vi "itc Hg box controller -- Pgg2.vi"(6 "Log File Path":path, 7 "itc box action":T8=enum."init", 8 "error in":errorcluster, 9 "Sweep Table In":dbl[][](array[numeric])=[[650.0, 1334.0, 30.0], [300.0, 1334.0, 0.0], [0.0, 0.0, 0.0], [0.0, 0.0, 0.0], [0.0, 0.0, 0.0], [0.0, 0.0, 0.0], [0.0, 0.0, 0.0], [0.0, 0.0, 0.0], [0.0, 0.0, 0.0], [0.0, 0.0, 0.0], [0.0, 0.0, 0.0], [300.0, 0.0, 0.0], [0.0, 0.0, 0.0], [0.0, 0.0, 0.0], [0.0, 0.0, 0.0], [300.0, 0.0, 0.0]], 10 "input":dbl=10.0, 11 "VISA resource name":refnum<visa-resource-name>="GPIB0::1::INSTR") -> (0 "error out":errorcluster, 1 "Sweep Table":dbl[][](array[numeric])=[[650.0, 1334.0, 30.0], [300.0, 1334.0, 0.0], [0.0, 0.0, 0.0], [0.0, 0.0, 0.0], [0.0, 0.0, 0.0], [0.0, 0.0, 0.0], [0.0, 0.0, 0.0], [0.0, 0.0, 0.0], [0.0, 0.0, 0.0], [0.0, 0.0, 0.0], [0.0, 0.0, 0.0], [300.0, 0.0, 0.0], [0.0, 0.0, 0.0], [0.0, 0.0, 0.0], [0.0, 0.0, 0.0], [300.0, 0.0, 0.0]], 2 "itc box state OUT":T7={"ITC503 Address"="GPIB0::15::INSTR", "ITC temperature"=0.0, "ITC set temperature"=300.0, "heater"=300.0, "gas flow"=1.6, "P"=0.0, "D"=10.0, "I"=0.1, "ITC state"="X0A1C2S01H1L0\r", "nonzero temperature"=0.0, "Magn Field (T)"=0.0})   [LabVIEW 2015]
uses:
  itc 503 box - control.ctl
  itc 503 box state.ctl
  mercury ixx/public/libraries/auxiliary/Controls/AUX Device (Set).ctl
  mercury ixx/public/libraries/auxiliary/Controls/AUX Signals (Set).ctl
  mercury ixx/public/libraries/auxiliary/Controls/AUX Device (Read).ctl
  mercury ixx/public/Controls/Manufacturing Data.ctl
  mercury ixx/public/libraries/auxiliary/Controls/AUX Signals (Read).ctl
  mercury ixx/public/Controls/ISOBus Address.ctl
  mercury ixx/public/Controls/Comms Transport Layer.ctl
  comparison control.ctl
  mercury ixx/public/Controls/Unit String.ctl
  mercury ixx/public/libraries/heater/Controls/Heater Device (Set).ctl
  mercury ixx/public/libraries/heater/Controls/Heater Signals Cluster.ctl
  Q - not nan -- real.vi
  mercury ixx/public/libraries/auxiliary/Open/Open Auxiliary Device.vi
  mercury ixx/public/libraries/auxiliary/configuration/Read/Aux Device (Read).vi
  mercury ixx/public/libraries/auxiliary/configuration/Set/Aux Device (Set).vi
  mercury ixx/public/libraries/Temperature/Open/Open Temperature Device.vi
  mercury ixx/public/libraries/Temperature/Configuration/Read/Temperature Device (Read).vi
  mercury ixx/public/libraries/control loop/configuration/Set/Temperature Setpoint (Set).vi
  mercury ixx/public/libraries/control loop/configuration/Set/P Value (Set).vi
  mercury ixx/public/libraries/control loop/configuration/Set/I Value (Set).vi
  mercury ixx/public/libraries/control loop/configuration/Set/D Value (Set).vi
  mercury ixx/public/libraries/control loop/configuration/Set/Heater Auto (Set).vi
  mercury ixx/public/libraries/heater/Open/Open Heater Device.vi
  mercury ixx/public/libraries/heater/Configuration/Read/Heater Device (Read).vi
  mercury ixx/public/libraries/heater/Configuration/Set/Heater Device (Set).vi
  mercury ixx/public/libraries/control loop/configuration/Read/Temperature Setpoint (Read).vi
  mercury ixx/public/libraries/control loop/configuration/Read/PID (Read).vi
  mercury ixx/public/libraries/heater/signals/Read/Voltage (Read).vi
  mercury ixx/public/libraries/System.lvlib
  mercury ixx/Mercury iXX.lvlib
  mercury ixx/public/libraries/Auxiliary.lvlib
  mercury ixx/public/libraries/Temperature.lvlib
  mercury ixx/public/libraries/Control Loop.lvlib
  mercury ixx/public/libraries/Heater.lvlib
panel:
  out "Tab Control":T1(tab)
  out "Auxiliary Device OUT":T2 {"Signals"."% Open" min=0.0 max=100.0 step=0.1 format="%.4f"; "Signals"."Position" max=20.0 step=1.0 format="%.4f"; "Speed" max=7 step=1; "Gear" max=7 step=1; "Temp V Err" min=0.0 max=20.0 step=0.1; "Temp Err" min=0.0 max=20.0 step=0.1; "Scaling Factor" min=0.0 max=99.0 step=0.1; "Min Flow" min=0.0 max=20.0 step=0.1}
  in  "Auxiliary Device IN":T5 {"Signals"."% Open" min=0.0 max=100.0 step=0.1 format="%#.1f"; "Speed" max=7 step=1; "Gear" max=7 step=1; "Temp V Err" min=0.0 max=20.0 step=0.1; "Temp Err" min=0.0 max=20.0 step=0.1; "Scaling Factor" min=0.0 max=99.0 step=0.1; "Min Flow" min=0.0 max=20.0 step=0.1}
  out "enabled state":enum16{"disabled", "enabled"}(ring)
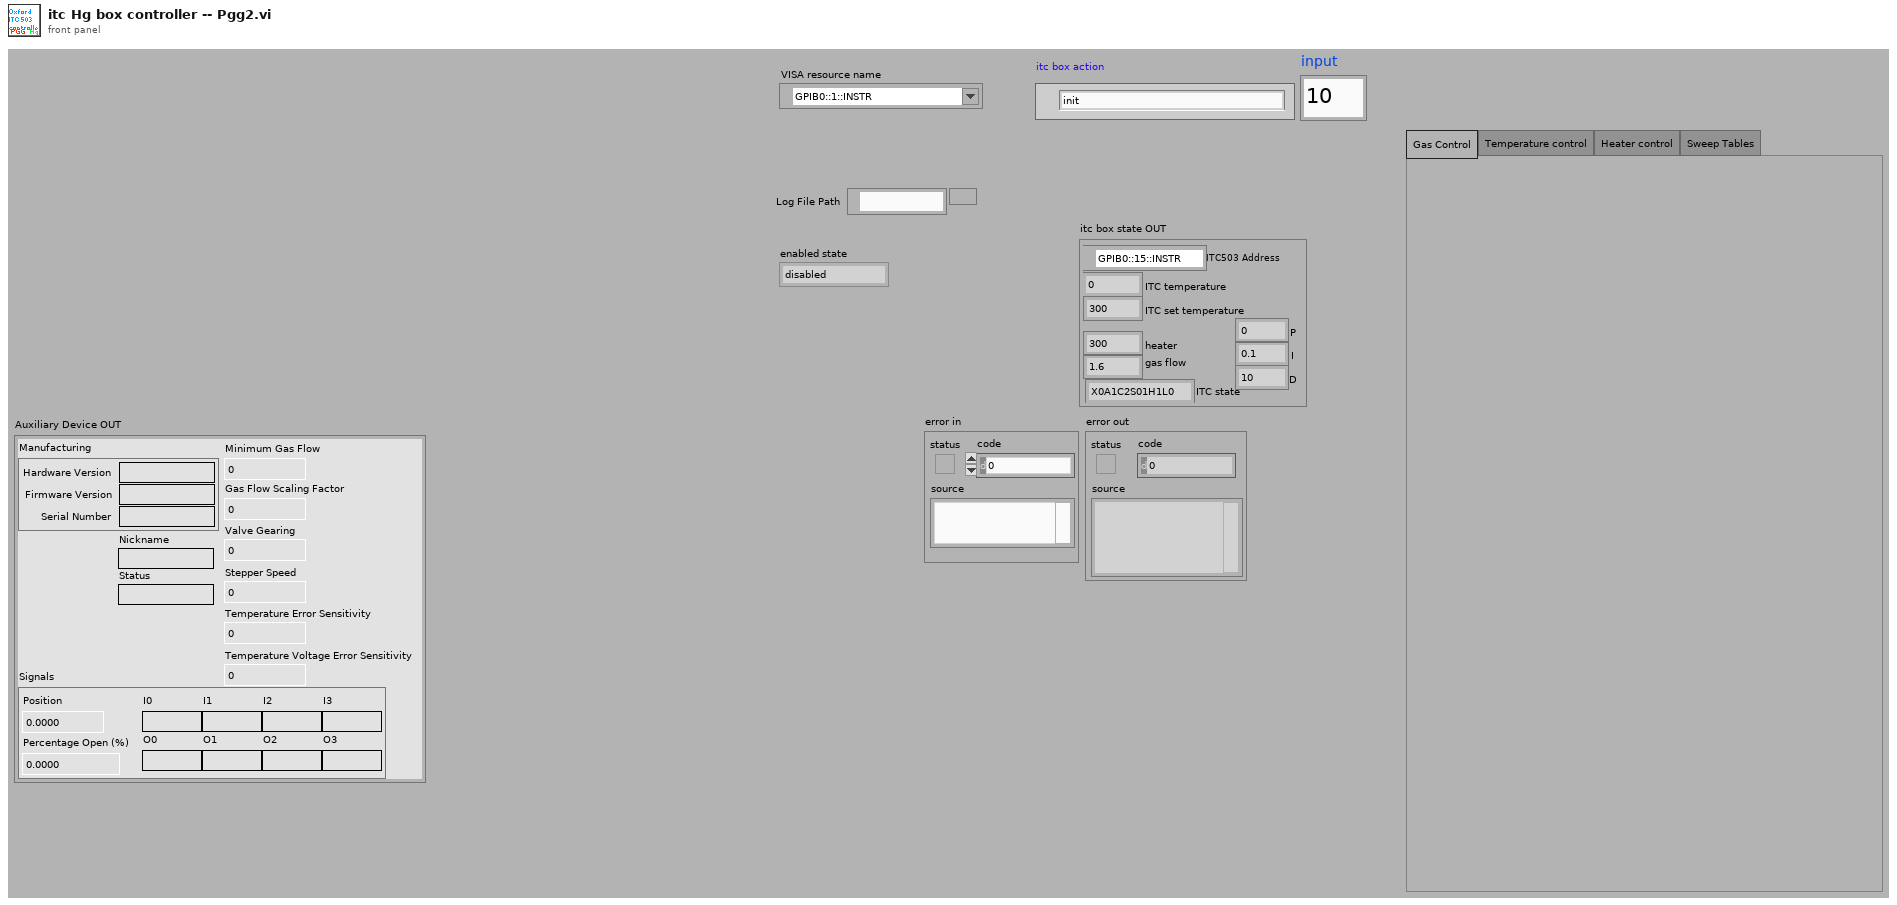
[diagram p1: front panel]
types:
  T1 = enum32{"Gas Control", "Temperature control", "Heater control", "Sweep Tables"}
  T2 = typedef "Mercury iXX.lvlib/Auxiliary.lvlib/AUX Device (Read).ctl" = cluster{"Manufacturing":T3, "Min Flow":dbl, "Scaling Factor":dbl, "Temp Err":dbl, "Temp V Err":dbl, "Gear":u32, "Speed":u32, "Signals":T4, "Nickname":string, "Status":string}
  T3 = typedef "Mercury iXX.lvlib/Manufacturing Data.ctl" = cluster{"Hardware Version":string, "Firmware Version":string, "Serial Number":string}
  T4 = typedef "Mercury iXX.lvlib/Auxiliary.lvlib/AUX Signals (Read).ctl" = cluster{"Position":dbl, "% Open":dbl, "I0":string, "I1":string, "I2":string, "I3":string, "O0":string, "O1":string, "O2":string, "O3":string}
  T5 = typedef "Mercury iXX.lvlib/Auxiliary.lvlib/AUX Device (Set).ctl" = cluster{"Min Flow":dbl, "Scaling Factor":dbl, "Temp Err":dbl, "Temp V Err":dbl, "Gear":u32, "Speed":u32, "Signals":T6}
  T6 = typedef "Mercury iXX.lvlib/Auxiliary.lvlib/AUX Signals (Set).ctl" = cluster{"% Open":dbl}
  T7 = typedef "itc 503 box state.ctl" = cluster{"ITC503 Address":refnum<visa-resource-name>, "ITC temperature":dbl, "ITC set temperature":dbl, "heater":dbl, "gas flow":dbl, "P":dbl, "D":dbl, "I":dbl, "ITC state":string, "nonzero temperature":dbl, "Magn Field (T)":dbl}
  T8 = typedef "itc 503 box - control.ctl" = enum16{"heater manual and zero", "heater auto", "upload D", "upload I", "upload P", "shut off", "init", "read sweep table", "disable", "enable", "read state", "set gas to", "stop sweep", "start sweep", "test", "set temperature to", "write sweep table", "-void", "set heater to"}
  T9 = typedef "Mercury iXX.lvlib/ISOBus Address.ctl" = i32
  T10 = typedef "Mercury iXX.lvlib/Comms Transport Layer.ctl" = enum16{"Ethernet TCP/IP", "USB", "ISOBus - RS-232", "GPIB"}
  T11 = typedef "Mercury iXX.lvlib/Unit String.ctl" = string
  T12 = typedef "Mercury iXX.lvlib/Heater.lvlib/Heater Device (Set).ctl" = cluster{"Nickname":string, "Voltage Limit":string, "Nominal Resistance":string, "Maximum Power":string, "Heater Signals":T13}
  T13 = typedef "Mercury iXX.lvlib/Heater.lvlib/Heater Signals Cluster.ctl" = cluster{"Voltage":string, "Current":string, "Power":string}
  T14 = typedef "Mercury iXX.lvlib/Mercury Reference.ctl" = cluster{"Comms":refnum<visa-resource-name>, "Device ID":string[], "Comms Layer":T10, "Command":string, "Query reference":T15}
  T15 = typedef "Mercury iXX.lvlib/Query Dynamic Reference.ctl" = refnum<vi>
  T16 = typedef "comparison control.ctl" = enum16{"not a number", "above", "in range", "below"}
  T17 = typedef "Mercury iXX.lvlib/Heater.lvlib/Heater Device (Read).ctl" = cluster{"Manufacturing":T3, "Nickname":string, "Voltage Limit":string, "Nominal Resistance":string, "Maximum Power":string, "Heater Signals":T13, "Status":string}
  T18 = typedef "Mercury iXX.lvlib/Control Loop.lvlib/PID cluster.ctl" = cluster{"P":dbl, "I":dbl, "D":dbl}
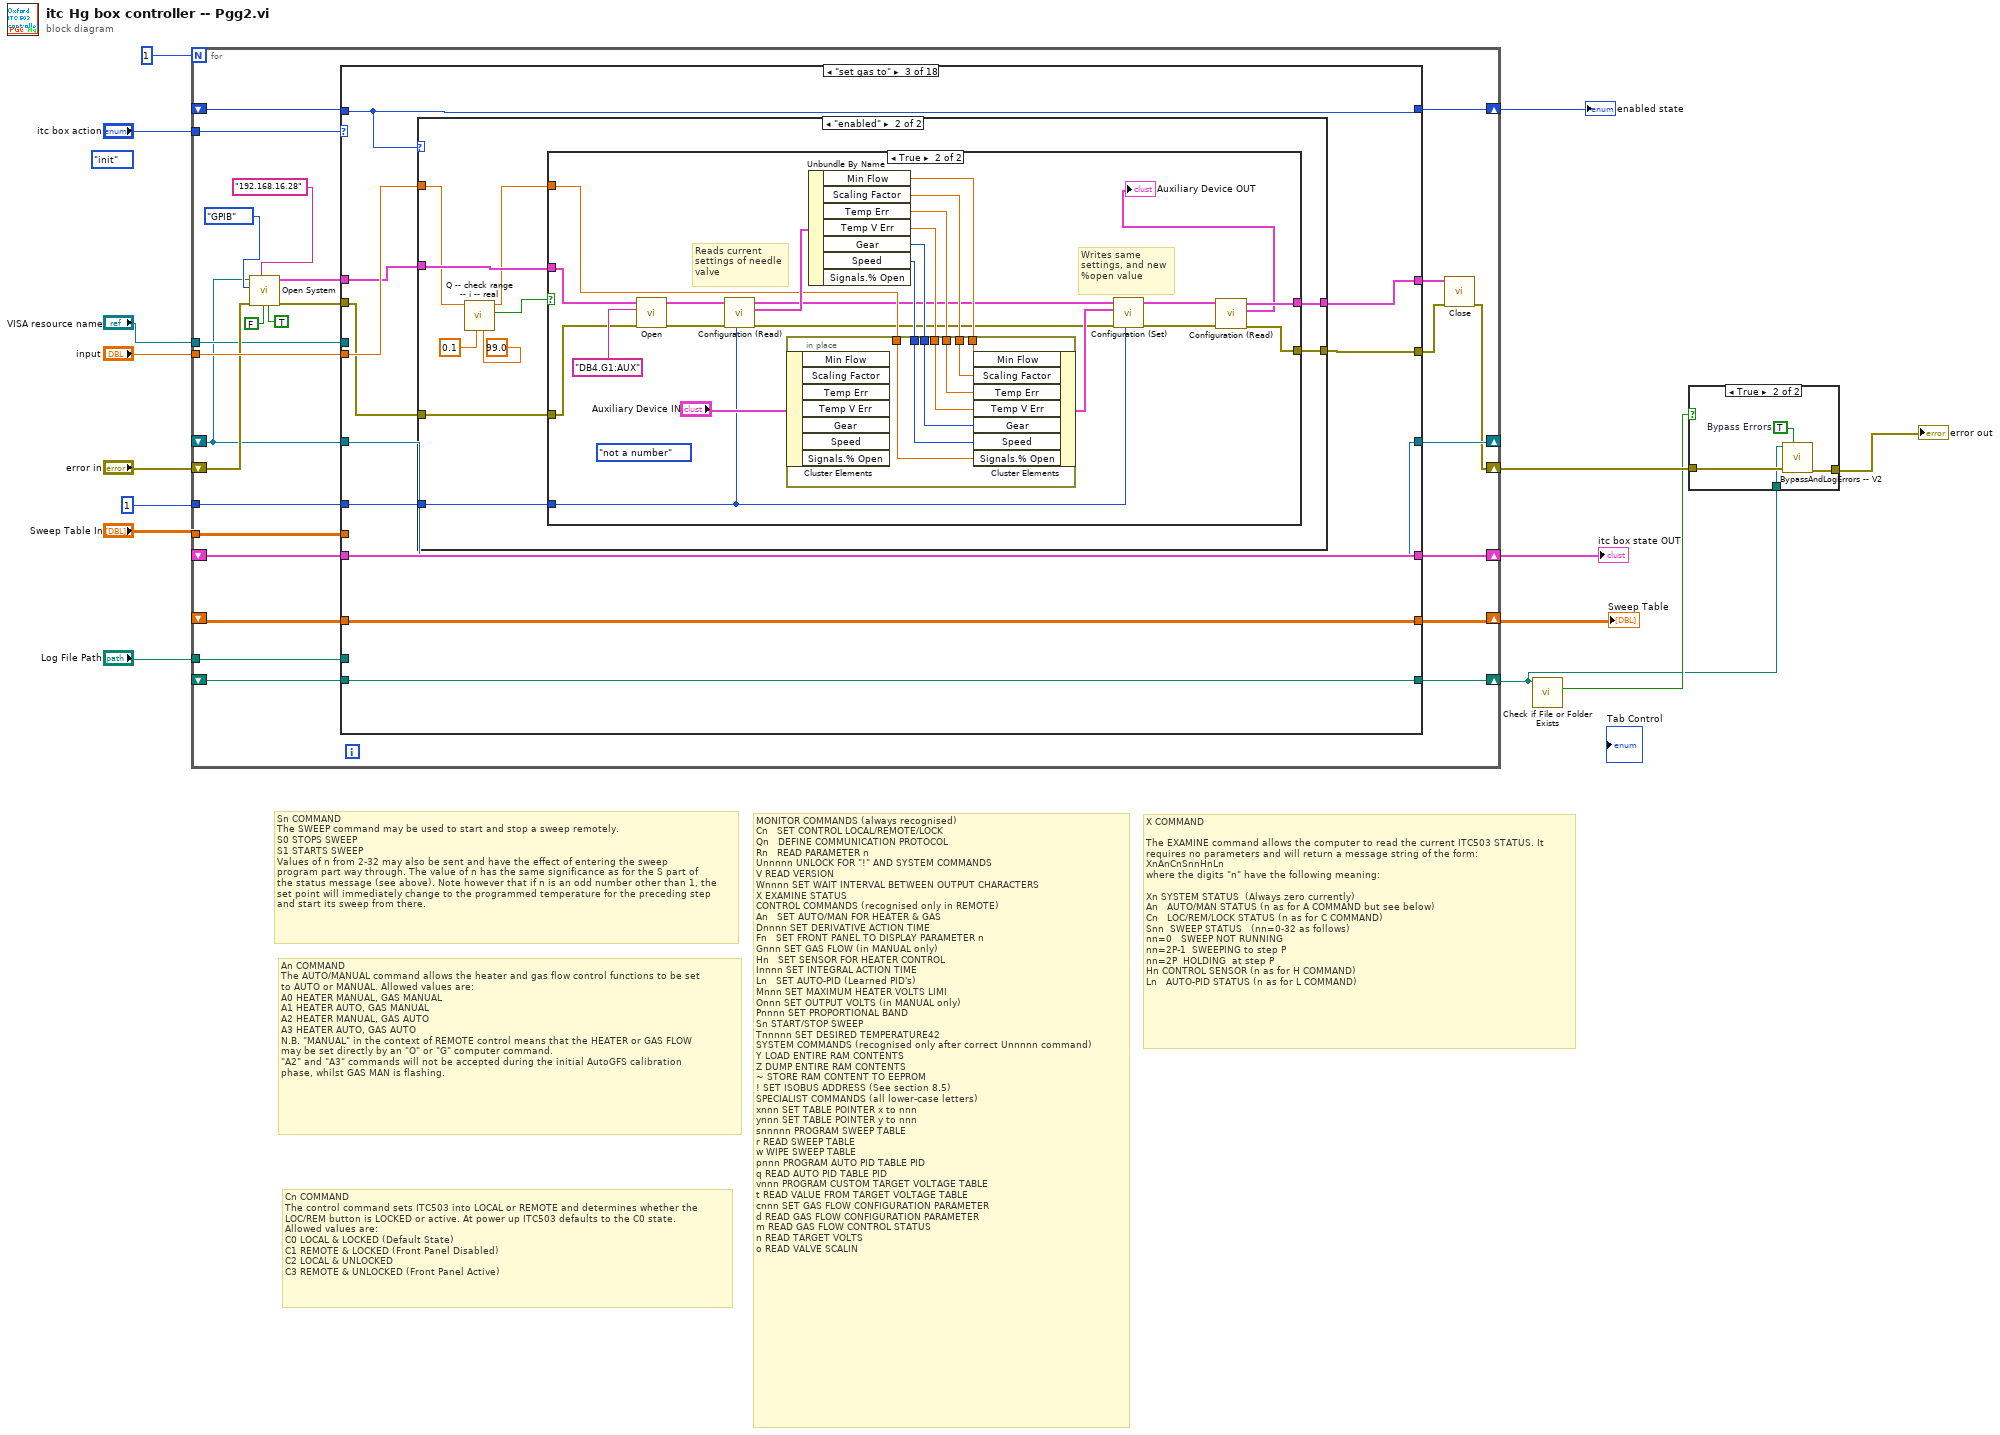
[diagram p0: block diagram]
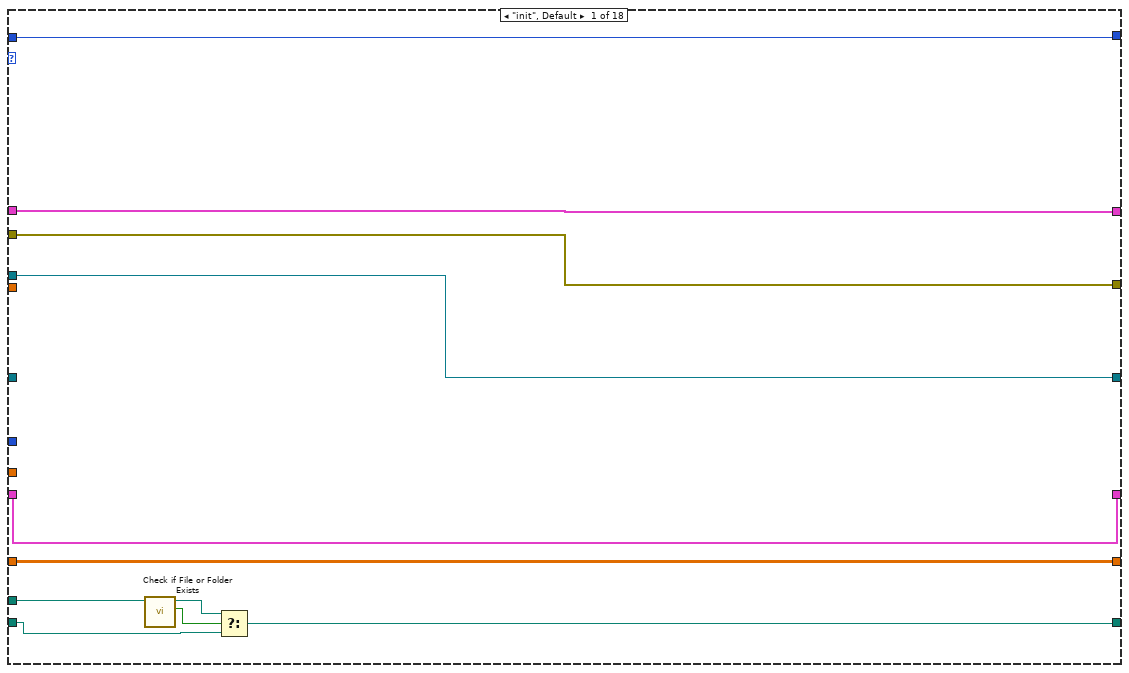
[diagram p3: hidden frame]
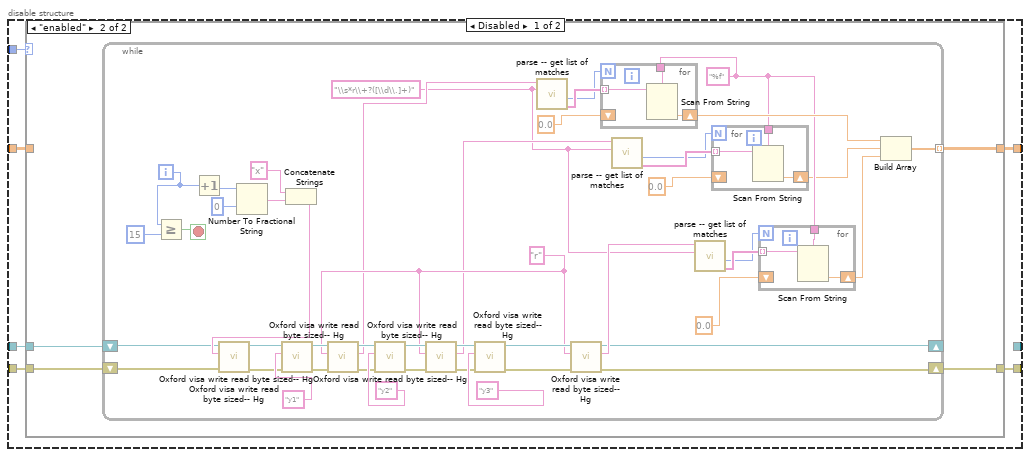
[diagram p5: hidden frame]
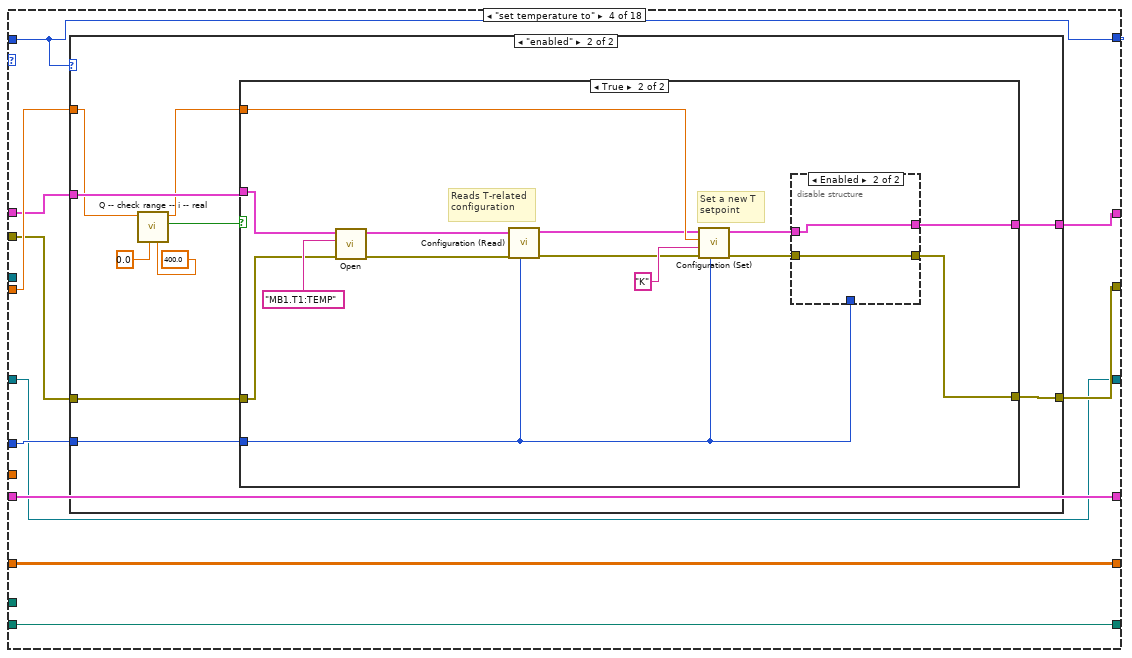
[diagram p9: hidden frame]
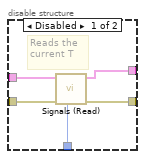
[diagram p12: hidden frame]
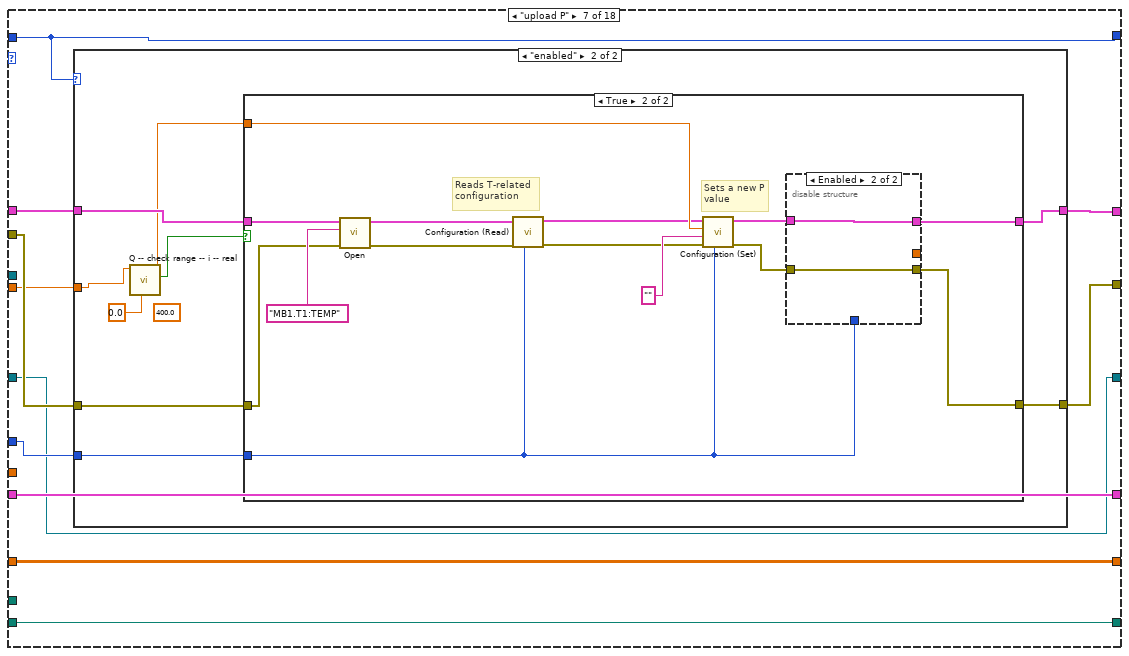
[diagram p15: hidden frame]
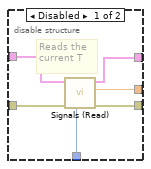
[diagram p18: hidden frame]
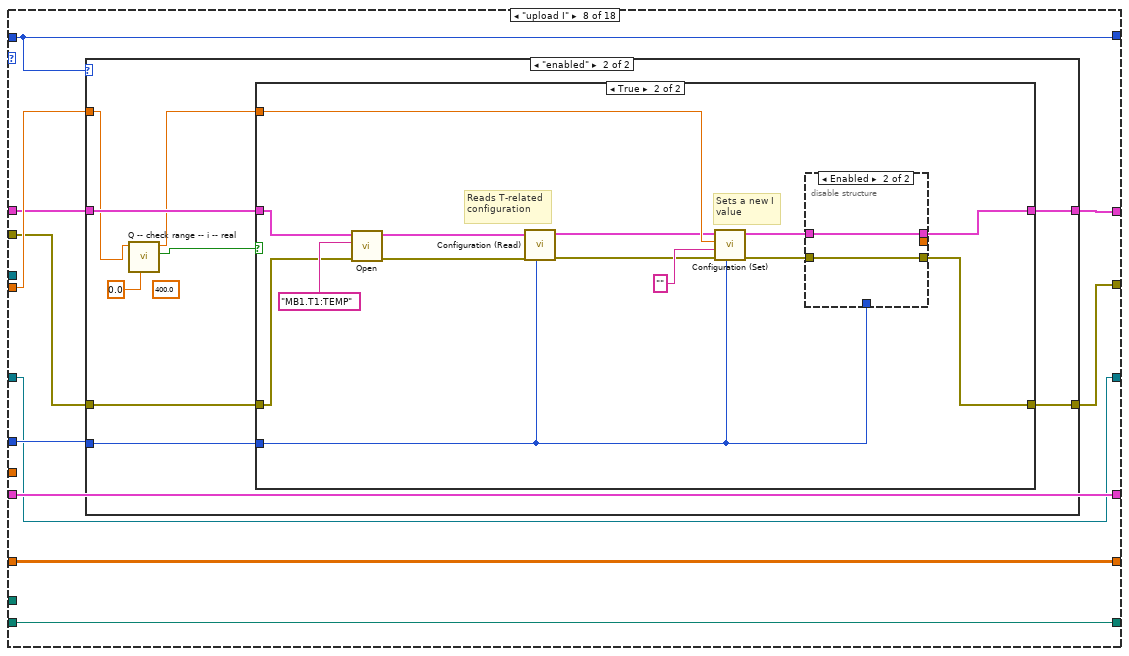
[diagram p19: hidden frame]
diagram:
  (unwired) itc_503_box_-_control."init" ("itc box action")
  # "Cn COMMAND\nThe control command sets ITC503 into LOCAL or REMOTE and determines whether the\nLOC/REM button is LOCKED or active. At power up ITC503 defaults to the C0 state.\nAllowed values are:\nC0 LOCAL & LOCKED (Default State)\nC1 REMOTE & LOCKED (Front Panel Disabled)\nC2 LOCAL & UNLOCKED\nC3 REMOTE & UNLOCKED (Front Panel Active)"
  # "An COMMAND\nThe AUTO/MANUAL command allows the heater and gas flow control functions to be set\nto AUTO or MANUAL. Allowed values are:\nA0 HEATER MANUAL, GAS MANUAL\nA1 HEATER AUTO, GAS MANUAL\nA2 HEATER MANUAL, GAS AUTO\nA3 HEATER AUTO, GAS AUTO\nN.B. \"MANUAL\" in the context of REMOTE control means that the HEATER or GAS FLOW\nmay be set directly by an \"O\" or \"G\" computer command.\n\"A2\" and \"A3\" commands will not be accepted during the initial AutoGFS calibration\nphase, whilst GAS MAN is flashing."
  # "MONITOR COMMANDS (always recognised)\nCn   SET CONTROL LOCAL/REMOTE/LOCK\nQn   DEFINE COMMUNICATION PROTOCOL\nRn   READ PARAMETER n\nUnnnnn UNLOCK FOR \"!\" AND SYSTEM COMMANDS\nV READ VERSION\nWnnnn SET WAIT INTERVAL BETWEEN OUTPUT CHARACTERS\nX EXAMINE STATUS\nCONTROL COMMANDS (recognised only in REMOTE)\nAn   SET AUTO/MAN FOR HEATER & GAS\nDnnnn SET DERIVATIVE ACTION TIME\nFn   SET FRONT PANEL TO DISPLAY PARAMETER n\nGnnn SET GAS FLOW (in MANUAL only)\nHn   SET SENSOR FOR HEATER CONTROL\nInnnn SET INTEGRAL ACTION TIME\nLn   SET AUTO-PID (Learned PID's)\nMnnn SET MAXIMUM HEATER VOLTS LIMI\nOnnn SET OUTPUT VOLTS (in MANUAL only)\nPnnnn SET PROPORTIONAL BAND\nSn START/STOP SWEEP\nTnnnnn SET DESIRED TEMPERATURE42\nSYSTEM COMMANDS (recognised only after correct Unnnnn command)\nY LOAD ENTIRE RAM CONTENTS\nZ DUMP ENTIRE RAM CONTENTS\n~ STORE RAM CONTENT TO EEPROM\n! SET ISOBUS ADDRESS (See section 8.5)\nSPECIALIST COMMANDS (all lower-case letters)\nxnnn SET TABLE POINTER x to nnn\nynnn SET TABLE POINTER y to nnn\nsnnnnn PROGRAM SWEEP TABLE\nr READ SWEEP TABLE\nw WIPE SWEEP TABLE\npnnn PROGRAM AUTO PID TABLE PID\nq READ AUTO PID TABLE PID\nvnnn PROGRAM CUSTOM TARGET VOLTAGE TABLE\nt READ VALUE FROM TARGET VOLTAGE TABLE\ncnnn SET GAS FLOW CONFIGURATION PARAMETER\nd READ GAS FLOW CONFIGURATION PARAMETER\nm READ GAS FLOW CONTROL STATUS\nn READ TARGET VOLTS\no READ VALVE SCALIN"
  # "X COMMAND\n\nThe EXAMINE command allows the computer to read the current ITC503 STATUS. It\nrequires no parameters and will return a message string of the form:\nXnAnCnSnnHnLn\nwhere the digits \"n\" have the following meaning:\n\nXn SYSTEM STATUS  (Always zero currently)\nAn   AUTO/MAN STATUS (n as for A COMMAND but see below)\nCn   LOC/REM/LOCK STATUS (n as for C COMMAND)\nSnn  SWEEP STATUS   (nn=0-32 as follows)\nnn=0   SWEEP NOT RUNNING\nnn=2P-1  SWEEPING to step P\nnn=2P  HOLDING  at step P\nHn CONTROL SENSOR (n as for H COMMAND)\nLn   AUTO-PID STATUS (n as for L COMMAND)"
  # "Sn COMMAND\nThe SWEEP command may be used to start and stop a sweep remotely.\nS0 STOPS SWEEP\nS1 STARTS SWEEP\nValues of n from 2-32 may also be sent and have the effect of entering the sweep\nprogram part way through. The value of n has the same significance as for the S part of\nthe status message (see above). Note however that if n is an odd number other than 1, the\nset point will immediately change to the programmed temperature for the preceding step\nand start its sweep from there."
  n1 = for {
    N: 1 -> [_]
    tunnel: "itc box action" -> [w41]
    shift-right: [w40] -> w10
    shift-left: _ -> [w39]
    shift-right: [w38] -> w13
    shift-left: _ -> [w37]
    tunnel: "input" -> [w36]
    tunnel: "Sweep Table In" -> [w35]
    tunnel: "Log File Path" -> [w34]
    shift-right: [w33] -> w1
    shift-left: _ -> [w32]
    tunnel: T9 1 ("ISOBUS address") -> [w31]
    shift-right: [w16] -> w6
    shift-left: "error in" -> [w26]
    shift-right: [w30] -> w7
    shift-left: _ -> [w29]
    shift-right: [w20] -> _
    shift-left: _ -> [w19]
    tunnel: "VISA resource name" -> [w21]
    n2 = call "Open System.vi"("Clear Previous Connections (False)"=TRUE, "ID Query (True)"=FALSE, "IP Address"="192.168.16.28", "error in (no error)"=w26, "Comms Layer"=Comms_Transport_Layer."GPIB", "VISA resource name"=w19) -> ("error out"=w25:errorcluster, "Mercury Reference Out"=w27:T14)  [unwired: 1 in, 3 out]
    n3 = case shown="\"set gas to\"" w41 {
      tunnel: [w43 w58 w139 w189 w238 w245 w255 w301 w341 w387 w427 w485 w551 w558 w565 w576 enum16{"disabled", "enabled"}."disabled" ("disable interaction with itc  2") enum16{"disabled", "enabled"}."enabled" ("disable interaction with itc  2")] -> w30
      tunnel: w29 -> [w43 w58 w139 w189 w238 w245 w255 w301 w341 w387 w427 w485 w551 w558 w565 w576 _ _]
      tunnel: [w52 w62 w143 w198 w240 w247 w258 w304 w350 w395 w433 w491 w553 w560 w567 w579 w631 w638] -> w40
      tunnel: w25 -> [w45 w60 w136 w191 w236 w243 w253 w298 w345 w388 w429 w488 w548 w557 w563 w578 w632 w639]
      tunnel: [w45 w59 w134 w194 w236 w243 w251 w296 w346 w391 w426 w483 w548 w557 w563 w577 w632 w639] -> w17
      tunnel: w39 -> [w52 w62 w143 w198 w240 w247 w258 w304 w350 w395 w433 w491 w553 w560 w567 w575 w631 w638]
      tunnel: [w51 w61 w142 w197 w239 w246 w257 w303 w349 w394 w432 w490 w552 w559 w566 w574 w630 w637] -> w38
      tunnel: w37 -> [w51 w57 w142 w197 w239 w246 w257 w303 w349 w394 w432 w490 w552 w559 w566 w574 w630 w637]
      tunnel: w36 -> [_ _ w138 w193 _ _ w252 w300 w342 _ _ w486 _ _ _ _ _ _]
      tunnel: w35 -> [_ _ _ _ _ _ _ _ _ _ _ _ _ _ _ _ _ _]
      tunnel: w34 -> [w50 _ _ _ _ _ _ _ _ _ _ _ _ _ _ _ _ _]
      tunnel: [w47 w56 w141 w196 w237 w244 w256 w302 w348 w393 w431 w489 w550 w556 w564 w573 w629 w636] -> w33
      tunnel: w32 -> [w46 w56 w141 w196 w237 w244 w256 w302 w348 w393 w431 w489 w550 w556 w564 w573 w629 w636]
      tunnel: [w44 w55 w135 w195 w235 w242 w249 w295 w347 w392 w425 w482 w549 w555 w562 w571 w628 w635] -> w18
      tunnel: w27 -> [w44 w55 w137 w192 w235 w242 w254 w299 w343 w390 w428 w487 w549 w555 w562 w572 w628 w635]
      tunnel: w31 -> [_ _ w140 w190 _ _ w250 w297 w344 w389 w430 w484 _ _ _ w570 _ _]
      tunnel: w21 -> [w42 _ _ _ _ _ _ _ _ _ _ _ _ _ _ _ _ _]
      tunnel: [w42 w53 w133 w188 w234 w241 w248 w294 w340 w386 w424 w481 w547 w554 w561 w568 w627 w634] -> w20
      tunnel: w19 -> [_ w54 w133 w188 w234 w241 w248 w294 w340 w386 w424 w481 w547 w554 w561 w569 w627 w634]
      frame "init", Default {
        n4 = call <vilib>:"Check if File or Folder Exists.vi"("path"=w50) -> ("file or folder exists?"=w49:bool, "dup path"=w48:path)  [unwired: 8 in, 1 out]
        n5 = Select(t=w48, s=w49, f=w46) -> (s? t:f=w47:path)
      }
      frame "read sweep table" {
        n6 = disable-structure shown="Enabled" {
          disable-tunnel: [w68 w132] -> w61
          disable-tunnel: w60 -> [w67 w131]
          disable-tunnel: [w66 w131] -> w59
          disable-tunnel: w58 -> [w65 _]
          disable-tunnel: w57 -> [w64 w132]
          disable-tunnel: w54 -> [w63 w130]
          disable-tunnel: [_ w130] -> w53
          frame Disabled {
            n7 = case shown="\"enabled\"" w65 {
              tunnel: [w69 w74] -> w68
              tunnel: w67 -> [w70 w73]
              tunnel: [w70 w72] -> w66
              tunnel: w64 -> [w69 _]
              tunnel: w63 -> [_ w71]
              frame "disabled", Default {
              }
              frame "enabled" {
                n8 = while {
                  tunnel: [w96] -> w74 mode=indexing
                  shift-right: [w76] -> _
                  shift-left: w71 -> [w99]
                  shift-right: [w75] -> w72
                  shift-left: w73 -> [w106]
                  i -> [w94]
                  stop <- w93 stop-if-true
                  w80 = "\\s*r\\+?([\\d\\.]+)" ("format string")
                  w79 = "%f" ("format string")
                  w98 = "r" ("string")
                  n9 = Greater Or Equal?(x=w94, y=15) -> (x >= y?=w93:bool)
                  n10 = Increment(x=w94) -> (x+1=w120:i32)
                  n11 = Number To Fractional String(number=w120, precision (6)=i16 0) -> (F-format string=w117:string)  [unwired: 2 in]
                  n12 = Concatenate Strings("x" ("string"), w117) -> (w116:string)
                  n13 = call "Oxford visa write read byte sized-- Hg.vi"("error in (no error)"=w106, "write buffer"=w116, "VISA resource name"=w99) -> ("error out"=w112:errorcluster, "VISA resource name out"=w100:refnum<visa-resource-name>)  [unwired: 6 in, 1 out]
                  n14 = call "Oxford visa write read byte sized-- Hg.vi"("error in (no error)"=w112, "write buffer"="y1" ("string"), "VISA resource name"=w100) -> ("error out"=w111:errorcluster, "VISA resource name out"=w101:refnum<visa-resource-name>)  [unwired: 6 in, 1 out]
                  n15 = call "Oxford visa write read byte sized-- Hg.vi"("error in (no error)"=w111, "write buffer"=w98, "VISA resource name"=w101) -> ("error out"=w110:errorcluster, "read buffer"=w92:string, "VISA resource name out"=w102:refnum<visa-resource-name>)  [unwired: 6 in]
                  n16 = call "Oxford visa write read byte sized-- Hg.vi"("error in (no error)"=w110, "write buffer"="y2" ("string"), "VISA resource name"=w102) -> ("error out"=w109:errorcluster, "VISA resource name out"=w105:refnum<visa-resource-name>)  [unwired: 6 in, 1 out]
                  n17 = call "Oxford visa write read byte sized-- Hg.vi"("error in (no error)"=w109, "write buffer"=w98, "VISA resource name"=w105) -> ("error out"=w108:errorcluster, "read buffer"=w81:string, "VISA resource name out"=w104:refnum<visa-resource-name>)  [unwired: 6 in]
                  n18 = call "Oxford visa write read byte sized-- Hg.vi"("error in (no error)"=w108, "write buffer"="y3" ("string"), "VISA resource name"=w104) -> ("error out"=w107:errorcluster, "VISA resource name out"=w103:refnum<visa-resource-name>)  [unwired: 6 in, 1 out]
                  n19 = call "parse -- get list of matches.vi"("regexp"=w80, "string"=w92) -> ("Array"=w91:string[], "number of free elastic constants"=w90:i32)  [unwired: 7 in, 1 out]
                  n20 = call "Oxford visa write read byte sized-- Hg.vi"("error in (no error)"=w107, "write buffer"=w98, "VISA resource name"=w103) -> ("error out"=w75:errorcluster, "read buffer"=w82:string, "VISA resource name out"=w76:refnum<visa-resource-name>)  [unwired: 6 in]
                  n21 = for {
                    N: w90 -> [_]
                    tunnel: w79 -> [w128]
                    tunnel: w91 -> [w127] mode=indexing
                    shift-right: [w129] -> w97
                    shift-left: 0.0 -> [_]
                    n22 = Scan From String(format string=w128, input string=w127) -> (output 1=w129:dbl)  [unwired: 3 in, 3 out]
                  }
                  n23 = call "parse -- get list of matches.vi"("regexp"=w80, "string"=w81) -> ("Array"=w88:string[], "number of free elastic constants"=w87:i32)  [unwired: 7 in, 1 out]
                  n24 = call "parse -- get list of matches.vi"("regexp"=w80, "string"=w82) -> ("Array"=w85:string[], "number of free elastic constants"=w84:i32)  [unwired: 7 in, 1 out]
                  n25 = for {
                    N: w87 -> [_]
                    tunnel: w88 -> [w125] mode=indexing
                    shift-right: [w126] -> w77
                    shift-left: 0.0 -> [_]
                    tunnel: w79 -> [w124]
                    n26 = Scan From String(format string=w124, input string=w125) -> (output 1=w126:dbl)  [unwired: 3 in, 3 out]
                  }
                  n27 = for {
                    N: w84 -> [_]
                    tunnel: w85 -> [w122] mode=indexing
                    shift-right: [w123] -> w78
                    shift-left: 0.0 -> [_]
                    tunnel: w79 -> [w121]
                    n28 = Scan From String(format string=w121, input string=w122) -> (output 1=w123:dbl)  [unwired: 3 in, 3 out]
                  }
                  n29 = Build Array(w97, w77, w78) -> (w96:dbl[])
                }
              }
            }
          }
          frame Enabled {
          }
        }
      }
      frame "set gas to" {
        n30 = case shown="\"enabled\"" w139 {
          tunnel: w138 -> [_ w149]
          tunnel: w136 -> [w145 w155]
          tunnel: [w145 w154] -> w134
          tunnel: w137 -> [w144 w153]
          tunnel: [w144 w152] -> w135
          tunnel: w140 -> [_ w151]
          frame "disabled", Default {
          }
          frame "enabled" {
            n31 = call "Q -- check range -- i -- real.vi"("upper"=99.0, "lower"=0.1 ("y"), "number"=w149) -> ("in range?"=w146:bool, "number in range"=w148:dbl)  [unwired: 6 in, 1 out]
            n32 = case shown="True" w146 {
              tunnel: w155 -> [w157 w178]
              tunnel: [w157 w160] -> w154
              tunnel: w148 -> [_ w166]
              tunnel: w153 -> [w156 w179]
              tunnel: [w156 w161] -> w152
              tunnel: w151 -> [_ w163]
              frame False {
              }
              frame True {
                (unwired) comparison_control."not a number" ("selector")
                # "Writes same settings, and new %open value"
                # "Reads current settings of needle valve"
                n33 = call-poly "Open.vi"("error in (no error)"=w178, "Device Identifier"="DB4.G1:AUX", "Mercury Reference In"=w179) -> ("error out"=w176:errorcluster, "Mercury Reference Out"=w177:T14)  [unwired: 7 out]
                n34 = call-poly "Configuration (Read).vi"("ISOBUS address"=w163, "error in"=w176, "Mercury Reference In"=w177) -> ("error out"=w164:errorcluster, "Auxiliary Device Details"=w175:T2, "Mercury Reference Out"=w165:T14)  [unwired: 6 out]
                n35 = Unbundle By Name(w175) -> ("Min Flow"=w172:dbl, "Scaling Factor"=w171:dbl, "Temp Err"=w170:dbl, "Temp V Err"=w169:dbl, "Gear"=w168:u32, "Speed"=w167:u32)  [unwired: 1 out]
                n36 = in-place {
                  in-place-border: w172 -> [w187]
                  in-place-border: w171 -> [w186]
                  in-place-border: w170 -> [w185]
                  in-place-border: w169 -> [w184]
                  in-place-border: w168 -> [w183]
                  in-place-border: w167 -> [w182]
                  in-place-border: w166 -> [w181]
                  n37 = in-place-cluster #1("Auxiliary Device IN") -> ()  [unwired: 7 out]
                  n38 = in-place-cluster #1("Min Flow"=w187, "Scaling Factor"=w186, "Temp Err"=w185, "Temp V Err"=w184, "Gear"=w183, "Speed"=w182, "Signals.% Open"=w181) -> (w173:T5)
                }
                n39 = call-poly "Configuration (Set).vi"("ISOBUS address"=w163, "error in"=w164, "Auxiliary Device"=w173, "Mercury Reference In"=w165) -> ("error out"=w159:errorcluster, "Mercury Reference Out"=w162:T14)  [unwired: 4 in, 2 out]
                n40 = call-poly "Configuration (Read).vi"("error in"=w159, "Mercury Reference In"=w162) -> ("error out"=w160:errorcluster, "Auxiliary Device Details"=→"Auxiliary Device OUT":T2, "Mercury Reference Out"=w161:T14)  [unwired: 1 in, 6 out]
              }
            }
          }
        }
      }
      frame "set temperature to" {
        n41 = case shown="\"enabled\"" w189 {
          tunnel: w193 -> [_ w204]
          tunnel: w191 -> [w200 w209]
          tunnel: [w200 w210] -> w194
          tunnel: w192 -> [w199 w206]
          tunnel: [w199 w208] -> w195
          tunnel: w190 -> [_ w207]
          frame "disabled", Default {
          }
          frame "enabled" {
            n42 = call "Q -- check range -- i -- real.vi"("upper"=400.0, "lower"=0.0 ("y"), "number"=w204) -> ("in range?"=w201:bool, "number in range"=w202:dbl)  [unwired: 6 in, 1 out]
            n43 = case shown="True" w201 {
              tunnel: [w212 w223] -> w210
              tunnel: w202 -> [_ w219]
              tunnel: w209 -> [w212 w224]
              tunnel: w206 -> [w211 w225]
              tunnel: [w211 w222] -> w208
              tunnel: w207 -> [_ w213]
              frame False {
              }
              frame True {
                # "Set a new T setpoint"
                # "Reads T-related configuration"
                n44 = call-poly "Open.vi"("error in (no error)"=w224, "Device Identifier"="MB1.T1:TEMP", "Mercury Reference In"=w225) -> ("error out"=w216:errorcluster, "Mercury Reference Out"=w217:T14)  [unwired: 7 out]
                n45 = call-poly "Configuration (Read).vi"("ISOBUS address"=w213, "error in"=w216, "Mercury Reference In"=w217) -> ("error out"=w215:errorcluster, "Mercury Reference Out"=w214:T14)  [unwired: 7 out]
                n46 = call-poly "Configuration (Set).vi"("ISOBUS address"=w213, "error in"=w215, "Unit"=T11 "K", "Temperature setpoint"=w219, "Mercury Reference In"=w214) -> ("error out"=w220:errorcluster, "Mercury Reference Out"=w221:T14)  [unwired: 3 in, 2 out]
                n47 = disable-structure shown="Enabled" {
                  disable-tunnel: [w231 w232] -> w223
                  disable-tunnel: [w230 w233] -> w222
                  disable-tunnel: w221 -> [w229 w233]
                  disable-tunnel: w220 -> [w228 w232]
                  disable-tunnel: w213 -> [w227 _]
                  frame Disabled {
                    # "Reads the current T"
                    n48 = call-poly "Signals (Read).vi"("ISOBUS address"=w227, "error in"=w228, "Mercury Reference In"=w229) -> ("error out"=w231:errorcluster, "Mercury Reference Out"=w230:T14)  [unwired: 7 out]
                  }
                  frame Enabled {
                  }
                }
              }
            }
          }
        }
      }
      frame "stop sweep" {
      }
      frame "start sweep" {
      }
      frame "upload P" {
        n49 = case shown="\"enabled\"" w255 {
          tunnel: w252 -> [_ w263]
          tunnel: w253 -> [w260 w268]
          tunnel: [w260 w269] -> w251
          tunnel: w254 -> [w259 w265]
          tunnel: [w259 w267] -> w249
          tunnel: w250 -> [_ w266]
          frame "disabled", Default {
          }
          frame "enabled" {
            (unwired) 400.0
            n50 = call "Q -- check range -- i -- real.vi"("lower"=0.0 ("y"), "number"=w263) -> ("in range?"=w262:bool, "number in range"=w261:dbl)  [unwired: 7 in, 1 out]
            n51 = case shown="True" w262 {
              tunnel: [w271 w282] -> w269
              tunnel: w261 -> [_ w278]
              tunnel: w268 -> [w271 w283]
              tunnel: w265 -> [w270 w284]
              tunnel: [w270 w281] -> w267
              tunnel: w266 -> [_ w272]
              frame False {
              }
              frame True {
                # "Sets a new P value"
                # "Reads T-related configuration"
                n52 = call-poly "Open.vi"("error in (no error)"=w283, "Device Identifier"="MB1.T1:TEMP", "Mercury Reference In"=w284) -> ("error out"=w275:errorcluster, "Mercury Reference Out"=w276:T14)  [unwired: 7 out]
                n53 = call-poly "Configuration (Read).vi"("ISOBUS address"=w272, "error in"=w275, "Mercury Reference In"=w276) -> ("error out"=w274:errorcluster, "Mercury Reference Out"=w273:T14)  [unwired: 7 out]
                n54 = call-poly "Configuration (Set).vi"("ISOBUS address"=w272, "error in"=w274, "Unit"=T11 "", "P Value"=w278, "Mercury Reference In"=w273) -> ("error out"=w279:errorcluster, "Mercury Reference Out"=w280:T14)  [unwired: 3 in, 2 out]
                n55 = disable-structure shown="Enabled" {
                  disable-tunnel: [w291 w292] -> w282
                  disable-tunnel: [w290 w293] -> w281
                  disable-tunnel: [w289 _] -> _
                  disable-tunnel: w280 -> [w288 w293]
                  disable-tunnel: w279 -> [w287 w292]
                  disable-tunnel: w272 -> [w286 _]
                  frame Disabled {
                    # "Reads the current T"
                    n56 = call-poly "Signals (Read).vi"("ISOBUS address"=w286, "error in"=w287, "Mercury Reference In"=w288) -> ("error out"=w291:errorcluster, "Temperature"=w289:dbl, "Mercury Reference Out"=w290:T14)  [unwired: 6 out]
                  }
                  frame Enabled {
                  }
                }
              }
            }
          }
        }
      }
      frame "upload I" {
        n57 = case shown="\"enabled\"" w301 {
          tunnel: w300 -> [_ w309]
          tunnel: w298 -> [w306 w314]
          tunnel: [w306 w315] -> w296
          tunnel: w299 -> [w305 w311]
          tunnel: [w305 w313] -> w295
          tunnel: w297 -> [_ w312]
          frame "disabled", Default {
          }
          frame "enabled" {
            (unwired) 400.0
            n58 = call "Q -- check range -- i -- real.vi"("lower"=0.0 ("y"), "number"=w309) -> ("in range?"=w307:bool, "number in range"=w308:dbl)  [unwired: 7 in, 1 out]
            n59 = case shown="True" w307 {
              tunnel: [w317 w328] -> w315
              tunnel: w308 -> [_ w324]
              tunnel: w314 -> [w317 w329]
              tunnel: w311 -> [w316 w330]
              tunnel: [w316 w327] -> w313
              tunnel: w312 -> [_ w318]
              frame False {
              }
              frame True {
                # "Sets a new I value"
                # "Reads T-related configuration"
                n60 = call-poly "Open.vi"("error in (no error)"=w329, "Device Identifier"="MB1.T1:TEMP", "Mercury Reference In"=w330) -> ("error out"=w321:errorcluster, "Mercury Reference Out"=w322:T14)  [unwired: 7 out]
                n61 = call-poly "Configuration (Read).vi"("ISOBUS address"=w318, "error in"=w321, "Mercury Reference In"=w322) -> ("error out"=w320:errorcluster, "Mercury Reference Out"=w319:T14)  [unwired: 7 out]
                n62 = call-poly "Configuration (Set).vi"("ISOBUS address"=w318, "error in"=w320, "Unit"=T11 "", "I Value"=w324, "Mercury Reference In"=w319) -> ("error out"=w325:errorcluster, "Mercury Reference Out"=w326:T14)  [unwired: 3 in, 2 out]
                n63 = disable-structure shown="Enabled" {
                  disable-tunnel: [w337 w338] -> w328
                  disable-tunnel: [w336 w339] -> w327
                  disable-tunnel: [w335 _] -> _
                  disable-tunnel: w326 -> [w334 w339]
                  disable-tunnel: w325 -> [w333 w338]
                  disable-tunnel: w318 -> [w332 _]
                  frame Disabled {
                    # "Reads the current T"
                    n64 = call-poly "Signals (Read).vi"("ISOBUS address"=w332, "error in"=w333, "Mercury Reference In"=w334) -> ("error out"=w337:errorcluster, "Temperature"=w335:dbl, "Mercury Reference Out"=w336:T14)  [unwired: 6 out]
                  }
                  frame Enabled {
                  }
                }
              }
            }
          }
        }
      }
      frame "upload D" {
        n65 = case shown="\"enabled\"" w341 {
          tunnel: w342 -> [_ w355]
          tunnel: w345 -> [w352 w360]
          tunnel: [w352 w361] -> w346
          tunnel: w343 -> [w351 w357]
          tunnel: [w351 w359] -> w347
          tunnel: w344 -> [_ w358]
          frame "disabled", Default {
          }
          frame "enabled" {
            (unwired) 400.0
            n66 = call "Q -- check range -- i -- real.vi"("lower"=0.0 ("y"), "number"=w355) -> ("in range?"=w353:bool, "number in range"=w354:dbl)  [unwired: 7 in, 1 out]
            n67 = case shown="True" w353 {
              tunnel: [w363 w374] -> w361
              tunnel: w354 -> [_ w370]
              tunnel: w360 -> [w363 w375]
              tunnel: w357 -> [w362 w376]
              tunnel: [w362 w373] -> w359
              tunnel: w358 -> [_ w364]
              frame False {
              }
              frame True {
                # "Sets a new D value"
                # "Reads T-related configuration"
                n68 = call-poly "Open.vi"("error in (no error)"=w375, "Device Identifier"="MB1.T1:TEMP", "Mercury Reference In"=w376) -> ("error out"=w367:errorcluster, "Mercury Reference Out"=w368:T14)  [unwired: 7 out]
                n69 = call-poly "Configuration (Read).vi"("ISOBUS address"=w364, "error in"=w367, "Mercury Reference In"=w368) -> ("error out"=w366:errorcluster, "Mercury Reference Out"=w365:T14)  [unwired: 7 out]
                n70 = call-poly "Configuration (Set).vi"("ISOBUS address"=w364, "error in"=w366, "Unit"=T11 "", "D Value"=w370, "Mercury Reference In"=w365) -> ("error out"=w371:errorcluster, "Mercury Reference Out"=w372:T14)  [unwired: 3 in, 2 out]
                n71 = disable-structure shown="Enabled" {
                  disable-tunnel: [w383 w384] -> w374
                  disable-tunnel: [w382 w385] -> w373
                  disable-tunnel: [w381 _] -> _
                  disable-tunnel: w372 -> [w380 w385]
                  disable-tunnel: w371 -> [w379 w384]
                  disable-tunnel: w364 -> [w378 _]
                  frame Disabled {
                    # "Reads the current T"
                    n72 = call-poly "Signals (Read).vi"("ISOBUS address"=w378, "error in"=w379, "Mercury Reference In"=w380) -> ("error out"=w383:errorcluster, "Temperature"=w381:dbl, "Mercury Reference Out"=w382:T14)  [unwired: 6 out]
                  }
                  frame Enabled {
                  }
                }
              }
            }
          }
        }
      }
      frame "heater auto" {
        n73 = case shown="\"enabled\"" w387 {
          tunnel: w388 -> [w397 w402]
          tunnel: [w397 w403] -> w391
          tunnel: w390 -> [w396 w399]
          tunnel: [w396 w401] -> w392
          tunnel: w389 -> [_ w400]
          frame "disabled", Default {
          }
          frame "enabled" {
            n74 = case shown="True" TRUE {
              tunnel: [w405 w409] -> w403
              tunnel: w402 -> [w405 w415]
              tunnel: w399 -> [w404 w416]
              tunnel: [w404 w408] -> w401
              tunnel: w400 -> [_ w407]
              frame False {
              }
              frame True {
                # "Heater Auto:\n1 to set to auto\n0 to set to manual"
                n75 = disable-structure shown="Enabled" {
                  disable-tunnel: w416 -> [w420 w423]
                  disable-tunnel: w415 -> [w419 w422]
                  disable-tunnel: [w418 w423] -> w413
                  disable-tunnel: [w417 w422] -> w412
                  frame Disabled {
                    n76 = call-poly "Open.vi"("error in (no error)"=w419, "Device Identifier"="MB0.H1:HTR", "Mercury Reference In"=w420) -> ("error out"=w417:errorcluster, "Mercury Reference Out"=w418:T14)  [unwired: 7 out]
                  }
                  frame Enabled {
                  }
                }
                n77 = call-poly "Open.vi"("error in (no error)"=w412, "Device Identifier"="MB1.T1:TEMP", "Mercury Reference In"=w413) -> ("error out"=w410:errorcluster, "Mercury Reference Out"=w411:T14)  [unwired: 7 out]
                n78 = call-poly "Configuration (Set).vi"("ISOBUS address"=w407, "error in"=w410, "Heater Auto"="1", "Mercury Reference In"=w411) -> ("error out"=w409:errorcluster, "Mercury Reference Out"=w408:T14)  [unwired: 4 in, 2 out]
              }
            }
          }
        }
      }
      frame "heater manual and zero" {
        n79 = case shown="\"enabled\"" w427 {
          tunnel: w429 -> [w435 w440]
          tunnel: [w435 w441] -> w426
          tunnel: w428 -> [w434 w439]
          tunnel: [w434 w438] -> w425
          tunnel: w430 -> [_ w437]
          frame "disabled", Default {
          }
          frame "enabled" {
            n80 = case shown="True" TRUE {
              tunnel: [w443 w459] -> w441
              tunnel: w440 -> [w443 w467]
              tunnel: w439 -> [w442 w468]
              tunnel: [w442 w458] -> w438
              tunnel: w437 -> [_ w455]
              frame False {
              }
              frame True {
                # "Heater Auto:\n1 to set to auto\n0 to set to manual"
                n81 = disable-structure shown="Enabled" {
                  disable-tunnel: w468 -> [w472 w475]
                  disable-tunnel: w467 -> [w471 w474]
                  disable-tunnel: [w470 w475] -> w457
                  disable-tunnel: [w469 w474] -> w456
                  frame Disabled {
                    n82 = call-poly "Open.vi"("error in (no error)"=w471, "Device Identifier"="MB0.H1:HTR", "Mercury Reference In"=w472) -> ("error out"=w469:errorcluster, "Mercury Reference Out"=w470:T14)  [unwired: 7 out]
                  }
                  frame Enabled {
                  }
                }
                n83 = call-poly "Open.vi"("error in (no error)"=w456, "Device Identifier"="MB1.T1:TEMP", "Mercury Reference In"=w457) -> ("error out"=w452:errorcluster, "Mercury Reference Out"=w453:T14)  [unwired: 7 out]
                n84 = call-poly "Configuration (Set).vi"("ISOBUS address"=w455, "error in"=w452, "Heater Auto"="0", "Mercury Reference In"=w453) -> ("error out"=w446:errorcluster, "Mercury Reference Out"=w449:T14)  [unwired: 4 in, 2 out]
                n85 = call-poly "Open.vi"("error in (no error)"=w446, "Device Identifier"="MB0.H1:HTR", "Mercury Reference In"=w449) -> ("error out"=w447:errorcluster, "Mercury Reference Out"=w448:T14)  [unwired: 7 out]
                n86 = call-poly "Configuration (Read).vi"("ISOBUS address"=w455, "error in"=w447, "Mercury Reference In"=w448) -> ("error out"=w465:errorcluster, "Device Details"=w445:T17, "Mercury Reference Out"=w464:T14)  [unwired: 6 out]
                n87 = Unbundle By Name(w445) -> ("Nickname"=w463:string, "Voltage Limit"=w462:string, "Nominal Resistance"=w461:string, "Maximum Power"=w460:string)
                n88 = in-place {
                  in-place-border: w463 -> [w480]
                  in-place-border: w462 -> [w479]
                  in-place-border: w461 -> [w478]
                  in-place-border: w460 -> [w477]
                  n89 = in-place-cluster #2(T12 {"Nickname"="", "Voltage Limit"="", "Nominal Resistance"="", "Maximum Power"="", "Heater Signals"={"Voltage"="", "Current"="", "Power"=""}} ("Heater Device Void")) -> ()  [unwired: 5 out]
                  n90 = in-place-cluster #2("Nickname"=w480, "Voltage Limit"=w479, "Nominal Resistance"=w478, "Maximum Power"=w477, "Heater Signals.Voltage"="0") -> (w466:T12)
                }
                n91 = call-poly "Configuration (Set).vi"("ISOBUS address"=w455, "error in"=w465, "Heater Device Settings"=w466, "Mercury Reference In"=w464) -> ("error out"=w459:errorcluster, "Mercury Reference Out"=w458:T14)  [unwired: 4 in, 2 out]
              }
            }
          }
        }
      }
      frame "set heater to" {
        n92 = case shown="\"enabled\"" w485 {
          tunnel: w486 -> [_ w496]
          tunnel: w488 -> [w493 w502]
          tunnel: [w493 w503] -> w483
          tunnel: w487 -> [w492 w501]
          tunnel: [w492 w500] -> w482
          tunnel: w484 -> [_ w499]
          frame "disabled", Default {
          }
          frame "enabled" {
            n93 = call "Q -- check range -- i -- real.vi"("upper"=39.0, "lower"=0.0 ("y"), "number"=w496) -> ("in range?"=w494:bool, "number in range"=w495:dbl)  [unwired: 6 in, 1 out]
            n94 = case shown="True" w494 {
              tunnel: [w505 w521] -> w503
              tunnel: w495 -> [_ w523]
              tunnel: w502 -> [w505 w533]
              tunnel: w501 -> [w504 w534]
              tunnel: [w504 w520] -> w500
              tunnel: w499 -> [_ w517]
              frame False {
              }
              frame True {
                # "Heater Auto:\n1 to set to auto\n0 to set to manual"
                n95 = disable-structure shown="Enabled" {
                  disable-tunnel: w534 -> [w538 w541]
                  disable-tunnel: w533 -> [w537 w540]
                  disable-tunnel: [w536 w541] -> w519
                  disable-tunnel: [w535 w540] -> w518
                  frame Disabled {
                    n96 = call-poly "Open.vi"("error in (no error)"=w537, "Device Identifier"="MB0.H1:HTR", "Mercury Reference In"=w538) -> ("error out"=w535:errorcluster, "Mercury Reference Out"=w536:T14)  [unwired: 7 out]
                  }
                  frame Enabled {
                  }
                }
                n97 = Number To Fractional String(number=w523, width (-)=i16 3, precision (6)=i16 4) -> (F-format string=w525:string)  [unwired: 1 in]
                n98 = call-poly "Open.vi"("error in (no error)"=w518, "Device Identifier"="MB1.T1:TEMP", "Mercury Reference In"=w519) -> ("error out"=w514:errorcluster, "Mercury Reference Out"=w515:T14)  [unwired: 7 out]
                n99 = call-poly "Configuration (Set).vi"("ISOBUS address"=w517, "error in"=w514, "Heater Auto"="0", "Mercury Reference In"=w515) -> ("error out"=w508:errorcluster, "Mercury Reference Out"=w511:T14)  [unwired: 4 in, 2 out]
                n100 = call-poly "Open.vi"("error in (no error)"=w508, "Device Identifier"="MB0.H1:HTR", "Mercury Reference In"=w511) -> ("error out"=w509:errorcluster, "Mercury Reference Out"=w510:T14)  [unwired: 7 out]
                n101 = call-poly "Configuration (Read).vi"("ISOBUS address"=w517, "error in"=w509, "Mercury Reference In"=w510) -> ("error out"=w531:errorcluster, "Device Details"=w507:T17, "Mercury Reference Out"=w530:T14)  [unwired: 6 out]
                n102 = Unbundle By Name(w507) -> ("Nickname"=w529:string, "Voltage Limit"=w528:string, "Nominal Resistance"=w527:string, "Maximum Power"=w526:string)
                n103 = in-place {
                  in-place-border: w529 -> [w546]
                  in-place-border: w528 -> [w545]
                  in-place-border: w527 -> [w544]
                  in-place-border: w526 -> [w543]
                  in-place-border: w525 -> [w542]
                  n104 = in-place-cluster #3(T12 {"Nickname"="", "Voltage Limit"="", "Nominal Resistance"="", "Maximum Power"="", "Heater Signals"={"Voltage"="", "Current"="", "Power"=""}} ("Heater Device Void")) -> ()  [unwired: 5 out]
                  n105 = in-place-cluster #3("Nickname"=w546, "Voltage Limit"=w545, "Nominal Resistance"=w544, "Maximum Power"=w543, "Heater Signals.Voltage"=w542) -> (w532:T12)
                }
                n106 = call-poly "Configuration (Set).vi"("ISOBUS address"=w517, "error in"=w531, "Heater Device Settings"=w532, "Mercury Reference In"=w530) -> ("error out"=w521:errorcluster, "Mercury Reference Out"=w520:T14)  [unwired: 4 in, 2 out]
              }
            }
          }
        }
      }
      frame "shut off" {
      }
      frame "test" {
      }
      frame "write sweep table" {
      }
      frame "read state" {
        n107 = case shown="\"enabled\"" w576 {
          tunnel: [w582 w622] -> w579
          tunnel: w578 -> [w583 w621]
          tunnel: [w583 w588] -> w577
          tunnel: w575 -> [w582 _]
          tunnel: w572 -> [w581 w594]
          tunnel: [w581 w587] -> w571
          tunnel: w570 -> [_ w584]
          tunnel: w569 -> [w580 w595]
          tunnel: [w580 w595] -> w568
          frame "disabled", Default {
          }
          frame "enabled" {
            n108 = call-poly "Open.vi"("error in (no error)"=w621, "Device Identifier"="MB1.T1:TEMP", "Mercury Reference In"=w594) -> ("error out"=w603:errorcluster, "Mercury Reference Out"=w604:T14)  [unwired: 7 out]
            n109 = call "Temperature (Read).vi"("ISOBUS address"=w584, "error in"=w603, "Mercury Reference In"=w604) -> ("error out"=w614:errorcluster, "Temperature"=w610:dbl, "Mercury Reference Out"=w613:T14)  [unwired: 4 in, 2 out]
            n110 = call-poly "Configuration (Read).vi"("ISOBUS address"=w584, "error in"=w614, "Mercury Reference In"=w613) -> ("error out"=w611:errorcluster, "Temperature Setpoint"=w609:dbl, "Mercury Reference Out"=w612:T14)  [unwired: 6 out]
            n111 = call-poly "Configuration (Read).vi"("ISOBUS address"=w584, "error in"=w611, "Mercury Reference In"=w612) -> ("error out"=w591:errorcluster, "PID"=w593:T18, "Mercury Reference Out"=w592:T14)  [unwired: 6 out]
            n112 = call "Heater Auto (Read).vi"("ISOBUS address"=w584, "error in"=w591, "Mercury Reference In"=w592) -> ("error out"=w589:errorcluster, "Heater Auto"=w586:string, "Mercury Reference Out"=w590:T14)  [unwired: 5 in, 1 out]
            n113 = call-poly "Open.vi"("error in (no error)"=w589, "Device Identifier"="DB4.G1:AUX", "Mercury Reference In"=w590) -> ("error out"=w619:errorcluster, "Mercury Reference Out"=w602:T14)  [unwired: 7 out]
            n114 = call-poly "Configuration (Read).vi"("ISOBUS address"=w584, "error in"=w619, "Mercury Reference In"=w602) -> ("error out"=w600:errorcluster, "Auxiliary Device Details"=w618:T2, "Mercury Reference Out"=w585:T14)  [unwired: 6 out]
            n115 = call-poly "Open.vi"("error in (no error)"=w600, "Device Identifier"="MB0.H1:HTR", "Mercury Reference In"=w585) -> ("error out"=w615:errorcluster, "Mercury Reference Out"=w616:T14)  [unwired: 7 out]
            n116 = call-poly "Signals (Read).vi"("ISOBUS address"=w584, "error in"=w615, "Mercury Reference In"=w616) -> ("error out"=w588:errorcluster, "Voltage"=w601:dbl, "Mercury Reference Out"=w587:T14)  [unwired: 6 out]
            n117 = Unbundle By Name(w618) -> ("Signals.% Open"=w605:dbl)
            n118 = Unbundle By Name(w593) -> ("P"=w608:dbl, "I"=w606:dbl, "D"=w607:dbl)
            n119 = case shown="\"OFF\", Default" w586 {
              tunnel: ["A0" "A1"] -> w599
              frame "OFF", Default {
              }
              frame "ON" {
              }
            }
            n120 = Concatenate Strings("X0", w599, "C2S00H0L0") -> (w597:string)
            n121 = Bundle By Name(cluster=T7 {"ITC503 Address"="GPIB0::15::INSTR", "ITC temperature"=0.0, "ITC set temperature"=0.0, "heater"=0.0, "gas flow"=0.0, "P"=0.0, "D"=0.0, "I"=0.0, "ITC state"="", "nonzero temperature"=0.0, "Magn Field (T)"=0.0} ("itc box state OUT"), "ITC503 Address"=w595, "ITC temperature"=w610, "ITC set temperature"=w609, "heater"=w601, "gas flow"=w605, "P"=w608, "D"=w607, "I"=w606, "ITC state"=w597) -> (w622:T7)
          }
        }
      }
      frame "disable" {
      }
      frame "enable" {
      }
    }
    n122 = call "Close.vi"("error in (no error)"=w17, "Mercury Reference"=w18) -> ("error out"=w16:errorcluster)  [unwired: 9 out]
  }
  "itc box state OUT" <- w10
  "Sweep Table" <- w13
  "enabled state" <- w7
  n123 = call <vilib>:"Check if File or Folder Exists.vi"("path"=w1) -> ("file or folder exists?"=w5:bool)  [unwired: 8 in, 2 out]
  n124 = case shown="True" w5 {
    tunnel: w6 -> [w641 w644]
    tunnel: [w641 w643] -> w4
    tunnel: w1 -> [_ w642]
    frame False {
    }
    frame True {
      w645 = TRUE  # Bypass Errors
      n125 = call "BypassAndLogErrors -- V2.vi"("Bypass Errors"=w645, "error in (no error)"=w644, "Log File Path"=w642) -> ("error out"=w643:errorcluster)  [unwired: 8 in]
    }
  }
  "error out" <- w4
